vi "Build Enum Array of each Item MERGE.vi"   [LabVIEW 2015]
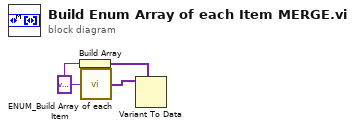
[diagram p0: block diagram]
diagram:
  w1 = variant ("Enum")
  n1 = Build Array(w1) -> (w3:variant[])
  n2 = call "ENUM_Build Array of each Item.vi"("Enum"=w1) -> ("Enum Array Out"=w2:variant[])  [unwired: 4 in]
  n3 = Variant To Data(type=w3, Variant=w2) -> ()  [unwired: 1 in, 2 out]
